vi "统计合格率.vi"() -> ()   [LabVIEW 2010]
uses:
  全局量/试验配置信息.vi
  全局量/自动测试结果.vi
  全局量/全局_配置.vi
panel:
  in  "自测序号":i32
  in  "LAN合格路数":i32
  in  "RS485合格路数":i32
  in  "RS232合格路数":i32
  in  "CAN合格路数":i32
  in  "模拟量AD合格路数":i32
  in  "模拟量DSP合格路数":i32
  in  "数字量输出合格路数":i32
  in  "数字量输入合格路数":i32
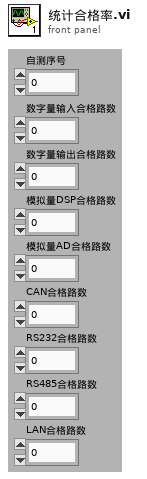
[diagram p1: front panel]
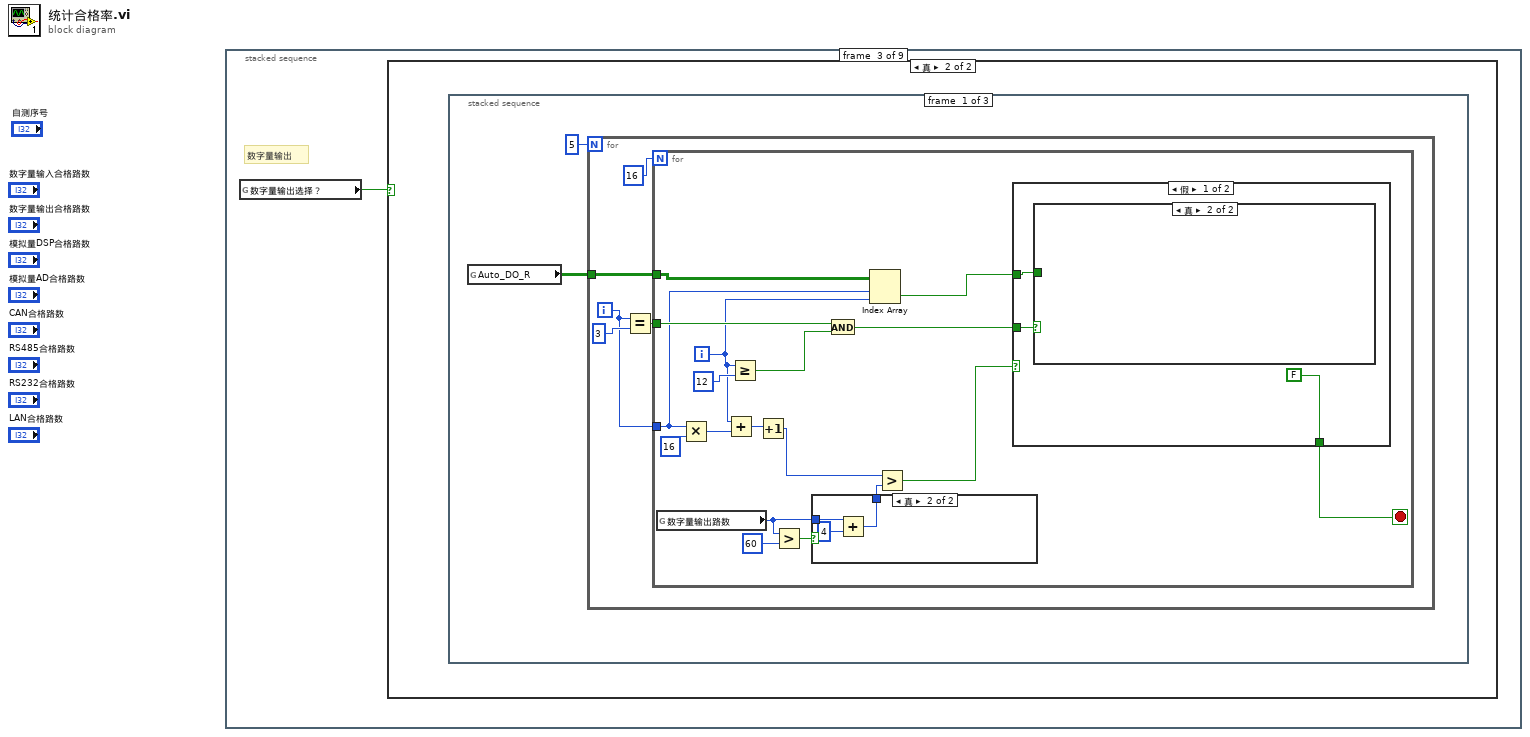
[diagram p0: block diagram]
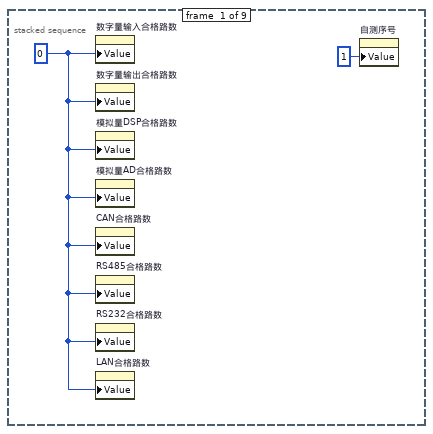
[diagram p2: hidden frame]
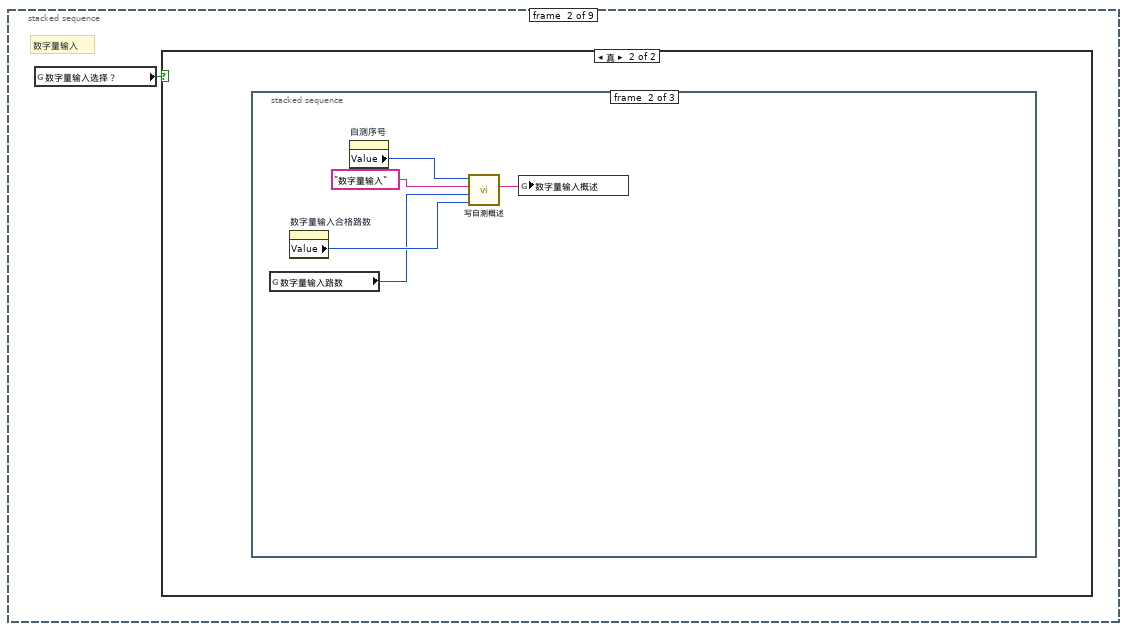
[diagram p3: hidden frame]
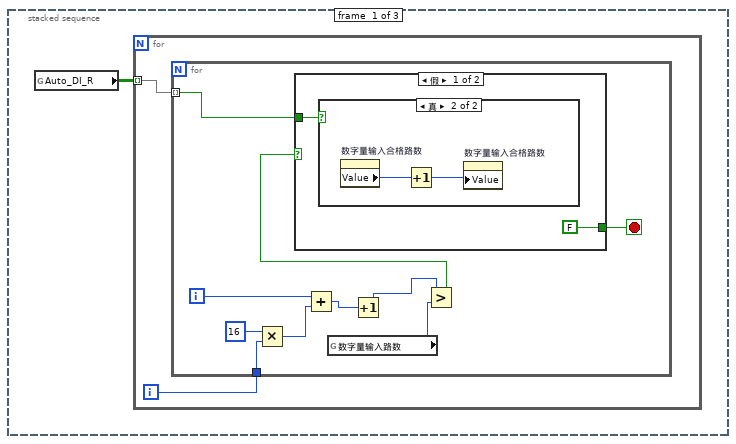
[diagram p5: hidden frame]
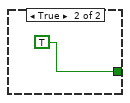
[diagram p7: hidden frame]
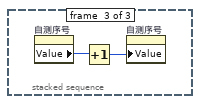
[diagram p8: hidden frame]
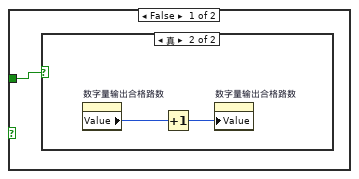
[diagram p10: hidden frame]
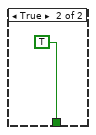
[diagram p12: hidden frame]
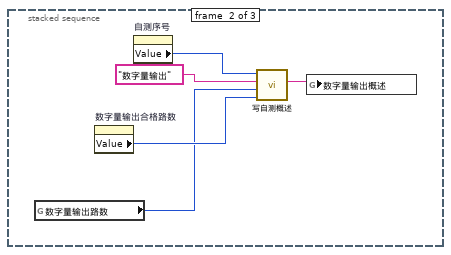
[diagram p14: hidden frame]
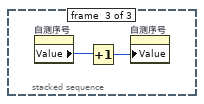
[diagram p15: hidden frame]
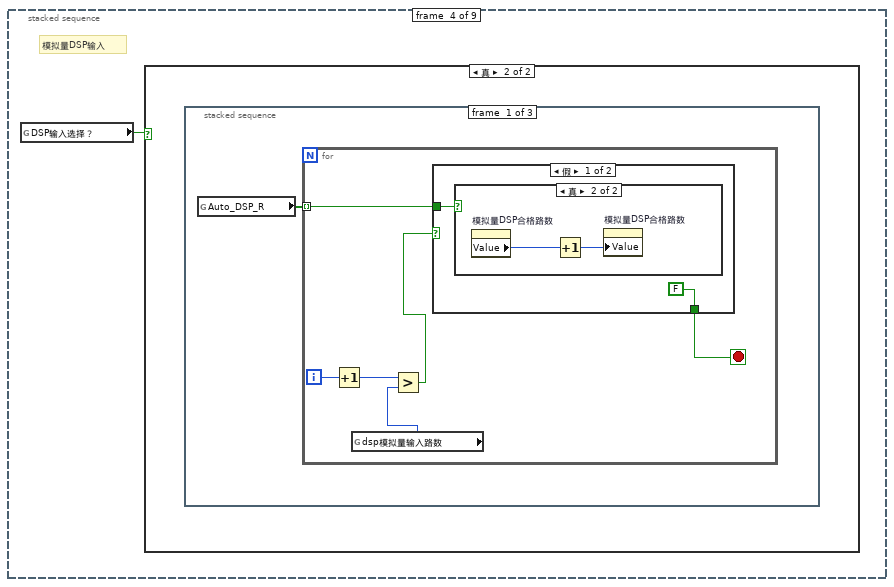
[diagram p16: hidden frame]
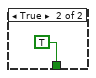
[diagram p19: hidden frame]
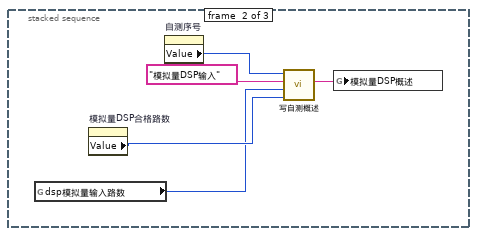
[diagram p20: hidden frame]
diagram:
  n1 = stacked-sequence {
    frame #0 {
      w2 = 0 ("数字量输入合格路数")
      n2 = property on="数字量输入合格路数" class="DigNum (严格)"("Value"=w2) -> ()  [unwired: 2 in, 2 out]
      n3 = property on="数字量输出合格路数" class="DigNum (严格)"("Value"=w2) -> ()  [unwired: 2 in, 2 out]
      n4 = property on="模拟量DSP合格路数" class="DigNum (严格)"("Value"=w2) -> ()  [unwired: 2 in, 2 out]
      n5 = property on="模拟量AD合格路数" class="DigNum (严格)"("Value"=w2) -> ()  [unwired: 2 in, 2 out]
      n6 = property on="CAN合格路数" class="DigNum (严格)"("Value"=w2) -> ()  [unwired: 2 in, 2 out]
      n7 = property on="RS485合格路数" class="DigNum (严格)"("Value"=w2) -> ()  [unwired: 2 in, 2 out]
      n8 = property on="RS232合格路数" class="DigNum (严格)"("Value"=w2) -> ()  [unwired: 2 in, 2 out]
      n9 = property on="LAN合格路数" class="DigNum (严格)"("Value"=w2) -> ()  [unwired: 2 in, 2 out]
      n10 = property on="自测序号" class="DigNum (严格)"("Value"=1 ("自测序号")) -> ()  [unwired: 2 in, 2 out]
    }
    frame #1 {
      # "数字量输入"
      n11 = global read "试验配置信息.vi" "数字量输入选择？"() -> (w3:bool)
      n12 = case shown="真" w3 {
        frame False {
        }
        frame True {
          n13 = stacked-sequence {
            frame #0 {
              n14 = global read "自动测试结果.vi" "Auto_DI_R"() -> (w4:bool[][])
              n15 = for {
                tunnel: w4 -> [w6] mode=indexing
                i -> [w5]
                n16 = for {
                  tunnel: w6 -> [w16] mode=indexing
                  tunnel: w5 -> [w15]
                  i -> [w12]
                  stop <- w7 stop-if-true
                  n17 = Multiply(x=16, y=w15) -> (x*y=w13:i32)
                  n18 = Add(x=w12, y=w13) -> (x+y=w11:i32)
                  n19 = global read "全局_配置.vi" "数字量输入路数"() -> (w9:i32)
                  n20 = Increment(x=w11) -> (x+1=w10:i32)
                  n21 = Greater?(x=w10, y=w9) -> (0:w8:bool)
                  n22 = case shown="假" w8 {
                    tunnel: w16 -> [w18 _]
                    tunnel: [FALSE TRUE] -> w7
                    frame False {
                      n23 = case shown="真" w18 {
                        frame False {
                        }
                        frame True {
                          n24 = property on="数字量输入合格路数" class="DigNum (严格)"() -> ("Value"=w19:i32)  [unwired: 2 in, 2 out]
                          n25 = Increment(x=w19) -> (x+1=w20:i32)
                          n26 = property on="数字量输入合格路数" class="DigNum (严格)"("Value"=w20) -> ()  [unwired: 2 in, 2 out]
                        }
                      }
                    }
                    frame True {
                    }
                  }
                }
              }
            }
            frame #1 {
              n27 = global read "全局_配置.vi" "数字量输入路数"() -> (w22:i32)
              n28 = property on="数字量输入合格路数" class="DigNum (严格)"() -> ("Value"=w24:i32)  [unwired: 2 in, 2 out]
              n29 = property on="自测序号" class="DigNum (严格)"() -> ("Value"=w26:i32)  [unwired: 2 in, 2 out]
              n30 = call "写自测概述.vi"("合格路数"=w24, "共路数"=w22, "测试事项"="数字量输入", "自测序号"=w26) -> ("概述字符串"=w23:string)  [unwired: 7 in]
              n31 = global write "自动测试结果.vi" "数字量输入概述"(w23) -> ()
            }
            frame #2 {
              n32 = property on="自测序号" class="DigNum (严格)"() -> ("Value"=w27:i32)  [unwired: 2 in, 2 out]
              n33 = Increment(x=w27) -> (x+1=w28:i32)
              n34 = property on="自测序号" class="DigNum (严格)"("Value"=w28) -> ()  [unwired: 2 in, 2 out]
            }
          }
        }
      }
    }
    frame #2 {
      # "数字量输出"
      n35 = global read "试验配置信息.vi" "数字量输出选择？"() -> (w29:bool)
      n36 = case shown="真" w29 {
        frame False {
        }
        frame True {
          n37 = stacked-sequence {
            frame #0 {
              n38 = global read "自动测试结果.vi" "Auto_DO_R"() -> (w31:bool[][])
              n39 = for {
                N: 5 -> [_]
                tunnel: w31 -> [w36]
                i -> [w33]
                n40 = Equal?(x=w33, y=3) -> (x = y?=w34:bool)
                n41 = for {
                  N: 16 -> [_]
                  tunnel: w36 -> [w44]
                  tunnel: w34 -> [w52]
                  tunnel: w33 -> [w42]
                  i -> [w41]
                  stop <- w45 stop-if-true
                  n42 = global read "全局_配置.vi" "数字量输出路数"() -> (w38:i32)
                  n43 = Multiply(x=w42, y=16) -> (x*y=w49:i32)
                  n44 = Add(x=w41, y=w49) -> (x+y=w48:i32)
                  n45 = Greater Or Equal?(x=w41, y=12) -> (x >= y?=w53:bool)
                  n46 = Increment(x=w48) -> (x+1=w47:i32)
                  n47 = Greater?(x=w38, y=60) -> (0:w39:bool)
                  n48 = case shown="真" w39 {
                    tunnel: w38 -> [w62 w65]
                    tunnel: [w62 w63] -> w37
                    frame False {
                    }
                    frame True {
                      n49 = Add(x=w65, y=4) -> (x+y=w63:i32)
                    }
                  }
                  n50 = And(x=w52, y=w53) -> (x .and. y?=w51:bool)
                  n51 = Index Array(array=w44, index (row)=w42, index (col)=w41) -> (element=w43:bool)
                  n52 = Greater?(x=w47, y=w37) -> (0:w46:bool)
                  n53 = case shown="假" w46 {
                    tunnel: w43 -> [w57 _]
                    tunnel: w51 -> [w56 _]
                    tunnel: [FALSE TRUE] -> w45
                    frame False {
                      n54 = case shown="真" w56 {
                        tunnel: w57 -> [w58 _]
                        frame False {
                          n55 = case shown="真" w58 {
                            frame False {
                            }
                            frame True {
                              n56 = property on="数字量输出合格路数" class="DigNum (严格)"() -> ("Value"=w59:i32)  [unwired: 2 in, 2 out]
                              n57 = Increment(x=w59) -> (x+1=w60:i32)
                              n58 = property on="数字量输出合格路数" class="DigNum (严格)"("Value"=w60) -> ()  [unwired: 2 in, 2 out]
                            }
                          }
                        }
                        frame True {
                        }
                      }
                    }
                    frame True {
                    }
                  }
                }
              }
            }
            frame #1 {
              n59 = global read "全局_配置.vi" "数字量输出路数"() -> (w66:i32)
              n60 = property on="数字量输出合格路数" class="DigNum (严格)"() -> ("Value"=w68:i32)  [unwired: 2 in, 2 out]
              n61 = property on="自测序号" class="DigNum (严格)"() -> ("Value"=w69:i32)  [unwired: 2 in, 2 out]
              n62 = call "写自测概述.vi"("合格路数"=w68, "共路数"=w66, "测试事项"="数字量输出", "自测序号"=w69) -> ("概述字符串"=w67:string)  [unwired: 7 in]
              n63 = global write "自动测试结果.vi" "数字量输出概述"(w67) -> ()
            }
            frame #2 {
              n64 = property on="自测序号" class="DigNum (严格)"() -> ("Value"=w72:i32)  [unwired: 2 in, 2 out]
              n65 = Increment(x=w72) -> (x+1=w71:i32)
              n66 = property on="自测序号" class="DigNum (严格)"("Value"=w71) -> ()  [unwired: 2 in, 2 out]
            }
          }
        }
      }
    }
    frame #3 {
      # "模拟量DSP输入"
      n67 = global read "试验配置信息.vi" "DSP输入选择？"() -> (w73:bool)
      n68 = case shown="真" w73 {
        frame False {
        }
        frame True {
          n69 = stacked-sequence {
            frame #0 {
              n70 = global read "自动测试结果.vi" "Auto_DSP_R"() -> (w74:bool[])
              n71 = for {
                tunnel: w74 -> [w80] mode=indexing
                i -> [w79]
                stop <- w75 stop-if-true
                n72 = Increment(x=w79) -> (x+1=w78:i32)
                n73 = global read "全局_配置.vi" "dsp模拟量输入路数"() -> (w77:u32)
                n74 = Greater?(x=w78, y=w77) -> (0:w76:bool)
                n75 = case shown="假" w76 {
                  tunnel: w80 -> [w82 _]
                  tunnel: [FALSE TRUE] -> w75
                  frame False {
                    n76 = case shown="真" w82 {
                      frame False {
                      }
                      frame True {
                        n77 = property on="模拟量DSP合格路数" class="DigNum (严格)"() -> ("Value"=w83:i32)  [unwired: 2 in, 2 out]
                        n78 = Increment(x=w83) -> (x+1=w84:i32)
                        n79 = property on="模拟量DSP合格路数" class="DigNum (严格)"("Value"=w84) -> ()  [unwired: 2 in, 2 out]
                      }
                    }
                  }
                  frame True {
                  }
                }
              }
            }
            frame #1 {
              n80 = global read "全局_配置.vi" "dsp模拟量输入路数"() -> (w86:u32)
              n81 = property on="模拟量DSP合格路数" class="DigNum (严格)"() -> ("Value"=w87:i32)  [unwired: 2 in, 2 out]
              n82 = property on="自测序号" class="DigNum (严格)"() -> ("Value"=w88:i32)  [unwired: 2 in, 2 out]
              n83 = call "写自测概述.vi"("合格路数"=w87, "共路数"=w86, "测试事项"="模拟量DSP输入", "自测序号"=w88) -> ("概述字符串"=w90:string)  [unwired: 7 in]
              n84 = global write "自动测试结果.vi" "模拟量DSP概述"(w90) -> ()
            }
            frame #2 {
              n85 = property on="自测序号" class="DigNum (严格)"() -> ("Value"=w91:i32)  [unwired: 2 in, 2 out]
              n86 = Increment(x=w91) -> (x+1=w92:i32)
              n87 = property on="自测序号" class="DigNum (严格)"("Value"=w92) -> ()  [unwired: 2 in, 2 out]
            }
          }
        }
      }
    }
    frame #4 {
      # "AD输入"
      n88 = global read "试验配置信息.vi" "AD输入选择？"() -> (w93:bool)
      n89 = case shown="真" w93 {
        frame False {
        }
        frame True {
          n90 = stacked-sequence {
            frame #0 {
              n91 = global read "自动测试结果.vi" "Auto_AD_R"() -> (w94:bool[])
              n92 = for {
                tunnel: w94 -> [w100] mode=indexing
                i -> [w99]
                stop <- w95 stop-if-true
                n93 = Increment(x=w99) -> (x+1=w97:i32)
                n94 = global read "全局_配置.vi" "ad模拟量输入路数"() -> (w98:u32)
                n95 = Greater?(x=w97, y=w98) -> (0:w96:bool)
                n96 = case shown="真" w96 {
                  tunnel: w100 -> [w102 _]
                  tunnel: [FALSE TRUE] -> w95
                  frame False {
                    n97 = case shown="真" w102 {
                      frame False {
                      }
                      frame True {
                        n98 = property on="模拟量AD合格路数" class="DigNum (严格)"() -> ("Value"=w104:i32)  [unwired: 2 in, 2 out]
                        n99 = Increment(x=w104) -> (x+1=w103:i32)
                        n100 = property on="模拟量AD合格路数" class="DigNum (严格)"("Value"=w103) -> ()  [unwired: 2 in, 2 out]
                      }
                    }
                  }
                  frame True {
                  }
                }
              }
            }
            frame #1 {
              n101 = global read "全局_配置.vi" "ad模拟量输入路数"() -> (w106:u32)
              n102 = property on="模拟量AD合格路数" class="DigNum (严格)"() -> ("Value"=w107:i32)  [unwired: 2 in, 2 out]
              n103 = property on="自测序号" class="DigNum (严格)"() -> ("Value"=w110:i32)  [unwired: 2 in, 2 out]
              n104 = call "写自测概述.vi"("合格路数"=w107, "共路数"=w106, "测试事项"="模拟量AD输入", "自测序号"=w110) -> ("概述字符串"=w108:string)  [unwired: 7 in]
              n105 = global write "自动测试结果.vi" "模拟量AD概述结果"(w108) -> ()
            }
            frame #2 {
              n106 = property on="自测序号" class="DigNum (严格)"() -> ("Value"=w111:i32)  [unwired: 2 in, 2 out]
              n107 = Increment(x=w111) -> (x+1=w112:i32)
              n108 = property on="自测序号" class="DigNum (严格)"("Value"=w112) -> ()  [unwired: 2 in, 2 out]
            }
          }
        }
      }
    }
    frame #5 {
      # "CAN总线测试"
      n109 = global read "试验配置信息.vi" "CAN选择？"() -> (w113:bool)
      n110 = case shown="真" w113 {
        frame False {
        }
        frame True {
          n111 = stacked-sequence {
            frame #0 {
              n112 = global read "自动测试结果.vi" "Auto_CAN_R"() -> (w114:bool[])
              n113 = for {
                tunnel: w114 -> [w120] mode=indexing
                i -> [w119]
                stop <- w115 stop-if-true
                n114 = Increment(x=w119) -> (x+1=w118:i32)
                n115 = global read "试验配置信息.vi" "自测CAN路数"() -> (w117:i32)
                n116 = Greater?(x=w118, y=w117) -> (0:w116:bool)
                n117 = case shown="真" w116 {
                  tunnel: w120 -> [w122 _]
                  tunnel: [FALSE TRUE] -> w115
                  frame False {
                    n118 = case shown="真" w122 {
                      frame False {
                      }
                      frame True {
                        n119 = property on="CAN合格路数" class="DigNum (严格)"() -> ("Value"=w124:i32)  [unwired: 2 in, 2 out]
                        n120 = Increment(x=w124) -> (x+1=w123:i32)
                        n121 = property on="CAN合格路数" class="DigNum (严格)"("Value"=w123) -> ()  [unwired: 2 in, 2 out]
                      }
                    }
                  }
                  frame True {
                  }
                }
              }
            }
            frame #1 {
              n122 = property on="CAN合格路数" class="DigNum (严格)"() -> ("Value"=w126:i32)  [unwired: 2 in, 2 out]
              n123 = global read "试验配置信息.vi" "自测CAN路数"() -> (w128:i32)
              n124 = property on="自测序号" class="DigNum (严格)"() -> ("Value"=w130:i32)  [unwired: 2 in, 2 out]
              n125 = call "写自测概述.vi"("合格路数"=w126, "共路数"=w128, "测试事项"="CAN通讯测试", "自测序号"=w130) -> ("概述字符串"=w127:string)  [unwired: 7 in]
              n126 = global write "自动测试结果.vi" "CAN测试概述"(w127) -> ()
            }
            frame #2 {
              n127 = property on="自测序号" class="DigNum (严格)"() -> ("Value"=w131:i32)  [unwired: 2 in, 2 out]
              n128 = Increment(x=w131) -> (x+1=w132:i32)
              n129 = property on="自测序号" class="DigNum (严格)"("Value"=w132) -> ()  [unwired: 2 in, 2 out]
            }
          }
        }
      }
    }
    frame #6 {
      # "RS232"
      n130 = global read "试验配置信息.vi" "RS232选择？"() -> (w133:bool)
      n131 = case shown="真" w133 {
        frame False {
        }
        frame True {
          n132 = stacked-sequence {
            frame #0 {
              n133 = global read "自动测试结果.vi" "Auto_RS232_R"() -> (w134:bool[])
              n134 = for {
                tunnel: w134 -> [w140] mode=indexing
                i -> [w139]
                stop <- w135 stop-if-true
                n135 = global read "全局_配置.vi" "R232路数"() -> (w138:u32)
                n136 = Increment(x=w139) -> (x+1=w137:i32)
                n137 = Greater?(x=w137, y=w138) -> (0:w136:bool)
                n138 = case shown="真" w136 {
                  tunnel: w140 -> [w142 _]
                  tunnel: [FALSE TRUE] -> w135
                  frame False {
                    n139 = case shown="真" w142 {
                      frame False {
                      }
                      frame True {
                        n140 = property on="RS232合格路数" class="DigNum (严格)"() -> ("Value"=w144:i32)  [unwired: 2 in, 2 out]
                        n141 = Increment(x=w144) -> (x+1=w143:i32)
                        n142 = property on="RS232合格路数" class="DigNum (严格)"("Value"=w143) -> ()  [unwired: 2 in, 2 out]
                      }
                    }
                  }
                  frame True {
                  }
                }
              }
            }
            frame #1 {
              n143 = global read "全局_配置.vi" "R232路数"() -> (w146:u32)
              n144 = property on="RS232合格路数" class="DigNum (严格)"() -> ("Value"=w147:i32)  [unwired: 2 in, 2 out]
              n145 = property on="自测序号" class="DigNum (严格)"() -> ("Value"=w150:i32)  [unwired: 2 in, 2 out]
              n146 = call "写自测概述.vi"("合格路数"=w147, "共路数"=w146, "测试事项"="串口RS232通讯", "自测序号"=w150) -> ("概述字符串"=w148:string)  [unwired: 7 in]
              n147 = global write "自动测试结果.vi" "串口RS232测试概述"(w148) -> ()
            }
            frame #2 {
              n148 = property on="自测序号" class="DigNum (严格)"() -> ("Value"=w151:i32)  [unwired: 2 in, 2 out]
              n149 = Increment(x=w151) -> (x+1=w152:i32)
              n150 = property on="自测序号" class="DigNum (严格)"("Value"=w152) -> ()  [unwired: 2 in, 2 out]
            }
          }
        }
      }
    }
    frame #7 {
      # "RS485"
      n151 = global read "试验配置信息.vi" "RS485选择？"() -> (w153:bool)
      n152 = case shown="真" w153 {
        frame False {
        }
        frame True {
          n153 = stacked-sequence {
            frame #0 {
              n154 = global read "自动测试结果.vi" "Auto_RS485_R"() -> (w154:bool[])
              n155 = for {
                tunnel: w154 -> [w155] mode=indexing
                n156 = case shown="真" w155 {
                  frame False {
                  }
                  frame True {
                    n157 = property on="RS485合格路数" class="DigNum (严格)"() -> ("Value"=w156:i32)  [unwired: 2 in, 2 out]
                    n158 = Increment(x=w156) -> (x+1=w157:i32)
                    n159 = property on="RS485合格路数" class="DigNum (严格)"("Value"=w157) -> ()  [unwired: 2 in, 2 out]
                  }
                }
              }
            }
            frame #1 {
              n160 = property on="RS485合格路数" class="DigNum (严格)"() -> ("Value"=w158:i32)  [unwired: 2 in, 2 out]
              n161 = global read "试验配置信息.vi" "自测485路数"() -> (w160:i32)
              n162 = property on="自测序号" class="DigNum (严格)"() -> ("Value"=w162:i32)  [unwired: 2 in, 2 out]
              n163 = call "写自测概述.vi"("合格路数"=w158, "共路数"=w160, "测试事项"="串口RS485通讯", "自测序号"=w162) -> ("概述字符串"=w159:string)  [unwired: 7 in]
              n164 = global write "自动测试结果.vi" "串口RS485测试概述"(w159) -> ()
            }
            frame #2 {
              n165 = property on="自测序号" class="DigNum (严格)"() -> ("Value"=w163:i32)  [unwired: 2 in, 2 out]
              n166 = Increment(x=w163) -> (x+1=w164:i32)
              n167 = property on="自测序号" class="DigNum (严格)"("Value"=w164) -> ()  [unwired: 2 in, 2 out]
            }
          }
        }
      }
    }
    frame #8 {
      # "LAN"
      n168 = global read "试验配置信息.vi" "LAN选择？"() -> (w165:bool)
      n169 = case shown="真" w165 {
        frame False {
        }
        frame True {
          n170 = stacked-sequence {
            frame #0 {
              n171 = global read "自动测试结果.vi" "Auto_LAN_R"() -> (w166:bool)
              n172 = case shown="真" w166 {
                frame False {
                }
                frame True {
                  n173 = property on="LAN合格路数" class="DigNum (严格)"() -> ("Value"=w168:i32)  [unwired: 2 in, 2 out]
                  n174 = Increment(x=w168) -> (x+1=w167:i32)
                  n175 = property on="LAN合格路数" class="DigNum (严格)"("Value"=w167) -> ()  [unwired: 2 in, 2 out]
                }
              }
            }
            frame #1 {
              n176 = global read "试验配置信息.vi" "自测LAN路数"() -> (w171:i32)
              n177 = property on="LAN合格路数" class="DigNum (严格)"() -> ("Value"=w169:i32)  [unwired: 2 in, 2 out]
              n178 = property on="自测序号" class="DigNum (严格)"() -> ("Value"=w173:i32)  [unwired: 2 in, 2 out]
              n179 = call "写自测概述.vi"("合格路数"=w169, "共路数"=w171, "测试事项"="以太网通讯测试", "自测序号"=w173) -> ("概述字符串"=w170:string)  [unwired: 7 in]
              n180 = global write "自动测试结果.vi" "以太网测试概述"(w170) -> ()
            }
            frame #2 {
              n181 = property on="自测序号" class="DigNum (严格)"() -> ("Value"=w174:i32)  [unwired: 2 in, 2 out]
              n182 = Increment(x=w174) -> (x+1=w175:i32)
              n183 = property on="自测序号" class="DigNum (严格)"("Value"=w175) -> ()  [unwired: 2 in, 2 out]
            }
          }
        }
      }
    }
  }
